vi "ep_Remove DC.vi"(5 "enable? (T)":bool=TRUE, 6 "IIR filter state in":cluster{"filter state":dbl[]}, 7 "reset? (F)":bool, 8 "error in (no error)":errorcluster, 9 "highpass IIR filter":T1={"filter structure"=enum."IIR 2nd Order", "Reverse Coefficients"=[-0.9998656982789184, 0.0, -1.9998656802413606, 0.999865698279524], "Forward Coefficients"=[0.9999328473978464, -1.9998656947956928, 0.9999328473978464, 0.9999328473978464, -0.9999328473978464, 0.0]}, 11 "signal in":dbl[](array[numeric])) -> (0 "error out":errorcluster, 3 "signal out":dbl[](array[numeric]), 4 "IIR filter state out":cluster{"filter state":dbl[]})   [LabVIEW 2014, in "NI_EP_Motor Monitoring.lvlib"]
uses:
  <vilib>/addons/Electrical Power/Motor Monitoring/NI_EP_Motor Monitoring.lvlib
  <vilib>/Analysis/3filter.llb/IIR Cascade Filter with I.C. (DBL).vi
  <vilib>/Analysis/NI_AALBase.lvlib
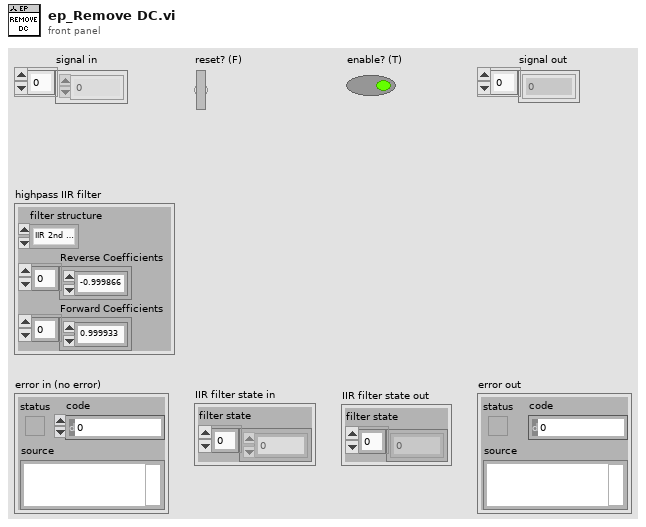
[diagram p1: front panel]
types:
  T1 = cluster{"filter structure":enum32{"IIR 2nd Order", "IIR 4th Order"}, "Reverse Coefficients":dbl[], "Forward Coefficients":dbl[]}
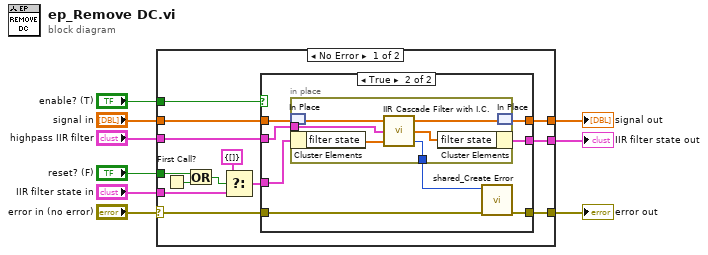
[diagram p0: block diagram]
diagram:
  n1 = case shown="No Error" "error in (no error)" {
    selector: "error in (no error)" -> [w18 w39]
    tunnel: "signal in" -> [w22 _]
    tunnel: "enable? (T)" -> [w21 _]
    tunnel: [w20 _] -> w7
    tunnel: "IIR filter state in" -> [w12 _]
    tunnel: "highpass IIR filter" -> [w19 _]
    tunnel: [w17 w39] -> w3
    tunnel: "reset? (F)" -> [w15 _]
    tunnel: [w10 _] -> w1
    frame No Error {
      n2 = First Call?() -> (First Call?: T/F=w16:bool)
      n3 = Or(x=w15, y=w16) -> (x .or. y?=w14:bool)
      n4 = Select(t=cluster{"filter state":dbl[]} {"filter state"=[]}, s=w14, f=w12) -> (s? t:f=w13:cluster{"filter state":dbl[]})
      n5 = case shown="True" w21 {
        tunnel: w22 -> [w24 w29]
        tunnel: [w24 w28] -> w20
        tunnel: w13 -> [_ w27]
        tunnel: w19 -> [_ w32]
        tunnel: w18 -> [w23 w31]
        tunnel: [w23 w30] -> w17
        tunnel: [_ w25] -> w10
        frame False {
        }
        frame True {
          n6 = in-place {
            in-place-border: w32 -> [w38]
            in-place-border: [w33] -> w26
            n7 = in-place-match #1(w29) -> (w37:dbl[])
            n8 = in-place-cluster #2(w27) -> ("filter state"=w35:dbl[])
            n9 = call-poly <vilib>:"IIR Cascade Filter with I.C..vi"("Initial Filter State"=w35, "IIR Filter Cluster"=w38, "X"=w37) -> ("error"=w33:i32, "Final Filter State"=w34:dbl[], "Filtered X"=w36:dbl[])
            n10 = in-place-cluster #2("filter state"=w34) -> (w25:cluster{"filter state":dbl[]})
            n11 = in-place-match #1(w36) -> (w28:dbl[])
          }
          n12 = call <vilib>:"shared_Create Error.vi"("error in (no error)"=w31, "error code (0)"=w26) -> ("error out"=w30:errorcluster)  [unwired: 9 in]
        }
      }
    }
    frame Error {
    }
  }
  "signal out" <- w7
  "error out" <- w3
  "IIR filter state out" <- w1
